vi "Get_Final_Path.vi"(8 "error in (no error)":errorcluster, 10 "AB_Build.lvclass":refnum<class "AB_Build.lvclass">, 11 "AB_Source in":refnum<class "AB_Source.lvclass">) -> (0 "error out":errorcluster, 3 "Final path":path)   [LabVIEW 2020, in "AB_Source.lvclass"]
uses:
  <vilib>/AppBuilder/AB_Classes/Source/AB_Source.lvclass
  <vilib>/AppBuilder/AB_Classes/Build/AB_Build.lvclass
  <vilib>/AppBuilder/AB_Classes/Source/AB_Source.lvclass/AB_Source.ctl
  <vilib>/AppBuilder/AB_Classes/Destination/AB_Destination.lvclass
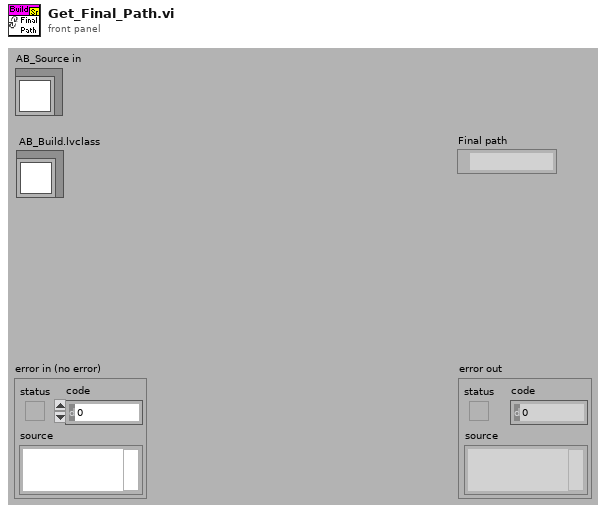
[diagram p1: front panel]
types:
  T1 = typedef "AB_Build.ctl" = cluster{"buildSpecName":string, "buildSpecDescription":string, "destinations":refnum<class "AB_Destination.lvclass">[], "exclusionOption":T2, "defaultLanguage":string, "supportedLanguages":string[], "excludedDirectories":path[], "buildContext":refnum<vi>, "buildObject":T3, "preview":bool, "programatic":bool, "progressBarEvents":T4, "userLog_Path":path, "preActionID":string, "preAction_Path":path, "postActionID":string, "postAction_Path":path, "eng_checkForBrokenVIs?":bool, "eng_verboseLinkerErrors?":bool, "localDest_Path":path, "targetDest_Path":path, "removeVIObject":u16, "cache":refnum<class "PreviewCache.lvclass">, "use cache":bool, "previewCache_ID":string, "buildCache_ID":string, "eng_TempLocalDest_Path":path, "eng_collectDependencies?":bool, "versionInfo":cluster{"buildVersion":cluster{"major":u16, "minor":u16, "patch":u16, "build":u16}, "autoIncrement":bool}, "eng_enableVIChecksums":bool}
  T2 = typedef "AB_Exclusion_Option.ctl" = cluster{"typedefs":bool, "polymorphicVIs":bool, "unusedLibraryItems":bool, "modifyLibraryFile":bool, "edit-timeDependencies":bool, "inlineVIs":bool, "dependent PPLs":bool, "dependent DLLs":bool}
  T3 = typedef "ItemRef.ctl" = u64
  T4 = typedef "provcom_ProgressBar_Events.ctl" = cluster{"newJob":refnum<user-event>, "newItem":refnum<user-event>, "errorMsg":T5, "cancel":refnum<user-event>}
  T5 = typedef "mxLvBuildError.ctl" = refnum<user-event>
  T6 = typedef "AB_Destination.ctl" = cluster{"destName":string, "path":path, "libraryName":string, "preserveHierarchy":bool, "eng_inBuild":bool, "eng_libraryReference":refnum<vi>, "eng_restictAddToNewLibrary":bool}
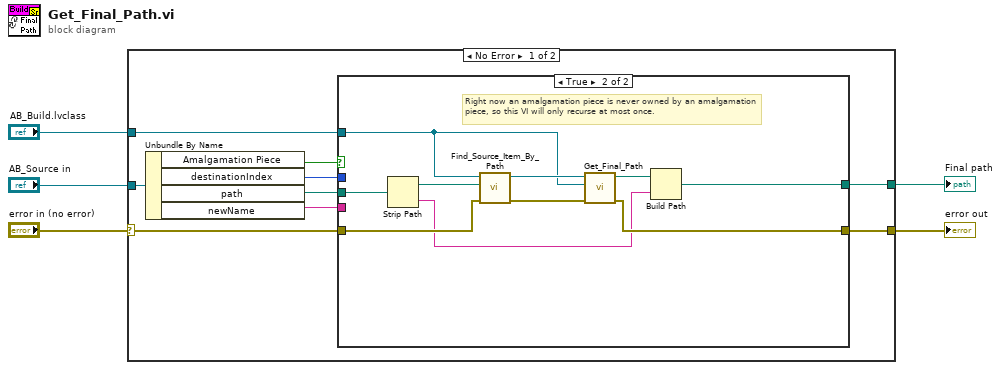
[diagram p0: block diagram]
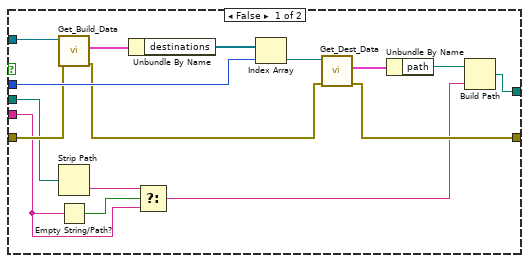
[diagram p2: hidden frame]
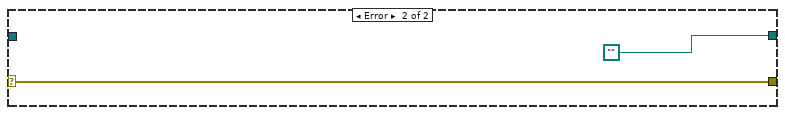
[diagram p3: hidden frame]
diagram:
  n1 = case shown="No Error" "error in (no error)" {
    selector: "error in (no error)" -> [w9 w41]
    tunnel: [w13 w41] -> w2
    tunnel: "AB_Source in" -> [w14 _]
    tunnel: "AB_Build.lvclass" -> [w6 _]
    tunnel: [w11 path "" ("appended path")] -> w5
    frame No Error {
      n2 = Unbundle By Name(w14) -> ("Amalgamation Piece"=w12:bool, "destinationIndex"=w10:i32, "path"=w7:path, "newName"=w8:string)
      n3 = case shown="True" w12 {
        tunnel: w7 -> [w17 w31]
        tunnel: w8 -> [w18 _]
        tunnel: w6 -> [w19 w35]
        tunnel: w9 -> [w24 w40]
        tunnel: w10 -> [w28 _]
        tunnel: [w29 w33] -> w11
        tunnel: [w30 w38] -> w13
        frame False {
          n4 = call <vilib>:"Get_Build_Data.vi"("error in (no error)"=w24, "Class in"=w19) -> ("error out"=w23:errorcluster, "data"=w20:T1)  [unwired: 7 in, 1 out]
          n5 = Strip Path(path=w17) -> (name=w16:string)  [unwired: 1 out]
          n6 = Empty String/Path?(string/path=w18) -> (empty?=w15:bool)
          n7 = Unbundle By Name(w20) -> ("destinations"=w21:refnum<class "AB_Destination.lvclass">[])
          n8 = Select(t=w16, s=w15, f=w18) -> (s? t:f=w27:string)
          n9 = Index Array(array=w21, index=w28) -> (element=w22:refnum<class "AB_Destination.lvclass">)
          n10 = call <vilib>:"Get_Dest_Data.vi"("error in (no error)"=w23, "Class in"=w22) -> ("error out"=w30:errorcluster, "destName"=w25:T6)  [unwired: 7 in, 1 out]
          n11 = Unbundle By Name(w25) -> ("path"=w26:path)
          n12 = Build Path(base path=w26, name or relative path=w27) -> (appended path=w29:path)
        }
        frame True {
          # "Right now an amalgamation piece is never owned by an amalgamation piece, so this VI will only recurse at most once."
          n13 = Strip Path(path=w31) -> (stripped path=w39:path, name=w32:string)
          n14 = call <vilib>:"Find_Source_Item_By_Path.vi"("error in (no error)"=w40, "Path"=w39, "AB_Build.lvclass"=w35) -> ("error out"=w34:errorcluster, "Found Source Item"=w36:refnum<class "AB_Source.lvclass">)  [unwired: 7 in]
          n15 = call-dynamic "Get_Final_Path.vi"("error in (no error)"=w34, "AB_Build.lvclass"=w35, "AB_Source in"=w36) -> ("error out"=w38:errorcluster, "Final path"=w37:path)  [unwired: 7 in]
          n16 = Build Path(base path=w37, name or relative path=w32) -> (appended path=w33:path)
        }
      }
    }
    frame Error {
    }
  }
  "error out" <- w2
  "Final path" <- w5
